vi "Inverse Rotate.vi"(0 "Position":i32, 1 "mV":u16, 2 "dir":bool, 3 "limit_mV":u16=2500, 4 "count_back":i32=2000) -> ()   [LabVIEW 2018]
panel:
  in  "stop":bool
  in  "temp":i32
  in  "Inv":bool
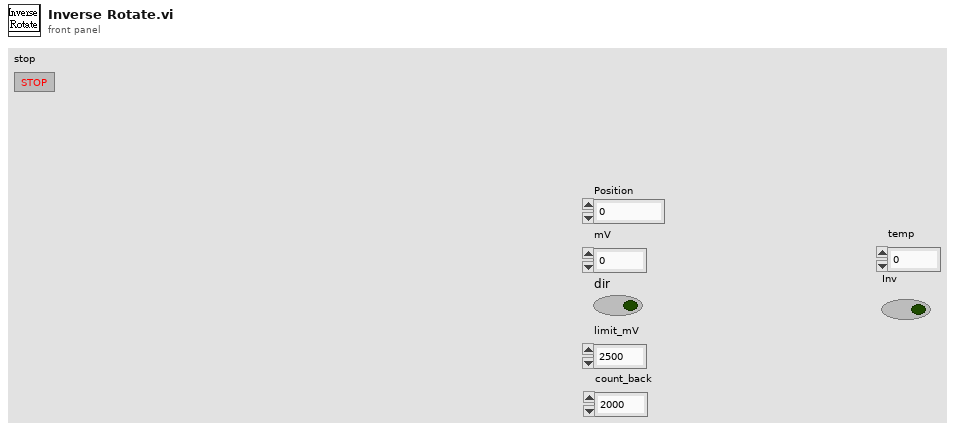
[diagram p1: front panel]
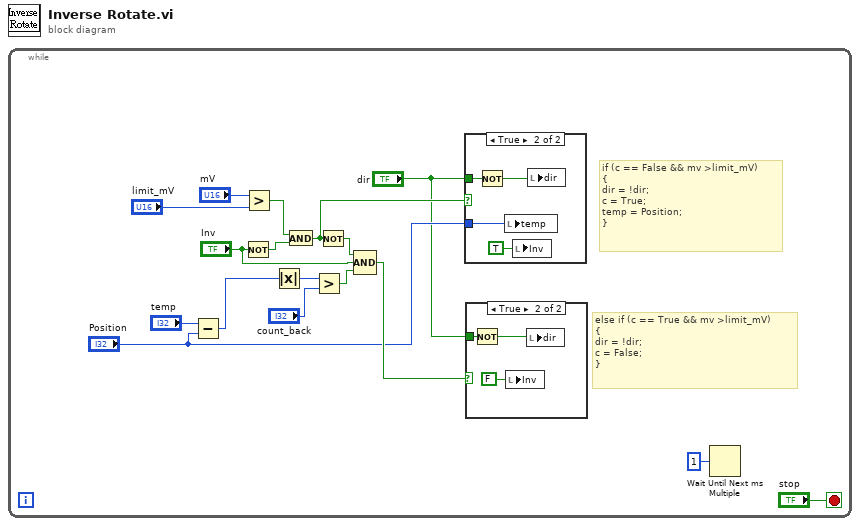
[diagram p0: block diagram]
diagram:
  n1 = while {
    stop <- "stop" stop-if-true
    # "else if (c == True && mv >limit_mV)\n{\ndir = !dir;\nc = False;\n}"
    # "if (c == False && mv >limit_mV)\n{\ndir = !dir;\nc = True;\ntemp = Position;\n}"
    n2 = Subtract(x="temp", y="Position") -> (x-y=w11:i32)
    n3 = Not(x="Inv") -> (.not. x?=w16:bool)
    n4 = Greater?(x="mV", y="limit_mV") -> (0:w17:bool)
    n5 = Absolute Value(x=w11) -> (abs(x)=w12:i32)
    n6 = And(x=w17, y=w16) -> (x .and. y?=w8:bool)
    n7 = Greater?(x=w12, y="count_back") -> (0:w13:bool)
    n8 = Not(x=w8) -> (.not. x?=w15:bool)
    n9 = Compound Arithmetic op=AND(w15, "Inv", w13) -> (w9:bool)
    n10 = case shown="True" w8 {
      tunnel: "dir" -> [_ w24]
      tunnel: "Position" -> [_ w23]
      frame False {
      }
      frame True {
        n11 = Not(x=w24) -> (.not. x?=w21:bool)
        n12 = local write "temp"(w23) -> ()
        n13 = local write "Inv"(TRUE ("Inv")) -> ()
        n14 = local write "dir"(w21) -> ()
      }
    }
    n15 = case shown="True" w9 {
      tunnel: "dir" -> [_ w20]
      frame False {
      }
      frame True {
        n16 = Not(x=w20) -> (.not. x?=w18:bool)
        n17 = local write "Inv"(FALSE ("Inv")) -> ()
        n18 = local write "dir"(w18) -> ()
      }
    }
    n19 = Wait Until Next ms Multiple(millisecond multiple=u32 1) -> ()  [unwired: 1 out]
  }
